vi "Set SMU1 Current Level 2.vi"(10 "N":i32) -> (2 "Smu1 current":dbl)   [LabVIEW 2010]
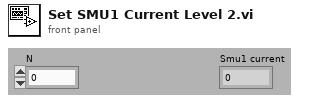
[diagram p1: front panel]
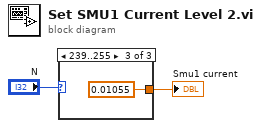
[diagram p0: block diagram]
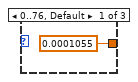
[diagram p2: hidden frame]
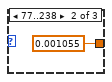
[diagram p3: hidden frame]
diagram:
  n1 = case shown="239..255" "N" {
    tunnel: [0.0001055 ("R 2") 0.001055 ("R 2") 0.01055 ("R 2")] -> w1
    frame 0..76, Default {
    }
    frame 77..238 {
    }
    frame 239..255 {
    }
  }
  "Smu1 current" <- w1
